vi "Functional Global.vi"(1 "FG Action (Read)":T1, 2 "var in":dbl) -> (0 "var out":dbl)   [LabVIEW 2009]
uses:
  cRIO/Functional Global Variables/Actions for FG's.ctl
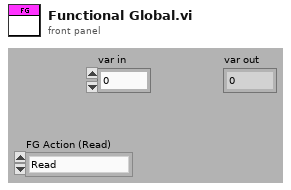
[diagram p1: front panel]
types:
  T1 = typedef "Actions for FG's.ctl" = enum16{"Read", "Write"}
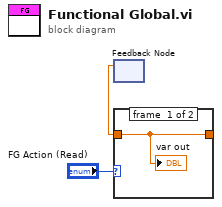
[diagram p0: block diagram]
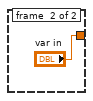
[diagram p2: hidden frame]
diagram:
  n1 = feedback #1() -> (w1:dbl)  [unwired: 1 in]
  n2 = case shown="\"Read\", Default" "FG Action (Read)" {
    tunnel: [w4 "var in"] -> w2
    tunnel: w1 -> [w4 _]
    frame #0 {
      "var out" <- w4
    }
    frame #1 {
    }
  }
